vi "ControlProgram.vi"() -> ()   [LabVIEW 2017]
uses:
  C:/Users/laserpc/Desktop/Luis Alarcon/StepByStep/Thorlabs.MotionControl.Controls.dll
  Thorlabs.MotionControl.Controls.dll
panel:
  in  "KCubeInertialMotorControl":refnum<k24>(container)
  in  "stop 2":bool
  in  "SerialNumber":string="97000098"
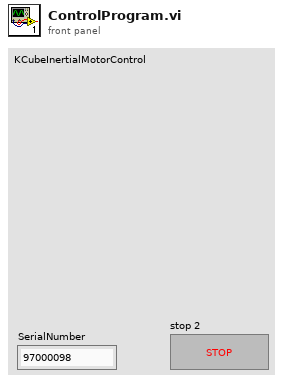
[diagram p1: front panel]
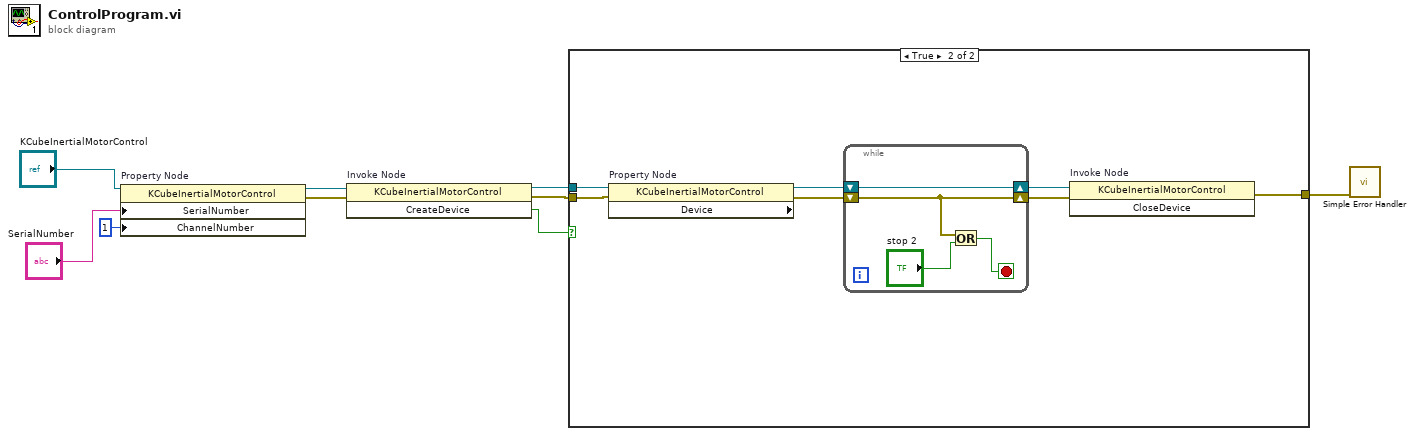
[diagram p0: block diagram]
diagram:
  n1 = property on="Property Node" class="KCubeInertialMotorControl"(reference="KCubeInertialMotorControl", "SerialNumber"="SerialNumber", "ChannelNumber"=1) -> (reference out=w8:refnum<k24>, error out=w5:errorcluster)  [unwired: 1 in]
  n2 = invoke on="Invoke Node" class="KCubeInertialMotorControl" method="CreateDevice"(reference=w8, error in=w5) -> (reference out=w7:refnum<k24>, error out=w2:errorcluster, "CreateDevice"=w3:bool)  [unwired: 1 in]
  n3 = case shown="True" w3 {
    tunnel: w7 -> [_ w17]
    tunnel: [w10 w16] -> w4
    tunnel: w2 -> [w10 w11]
    frame False {
    }
    frame True {
      n4 = property on="Property Node" class="KCubeInertialMotorControl" props=["Device"](reference=w17, error in=w11) -> (reference out=w15:refnum<k24>, error out=w14:errorcluster)  [unwired: 1 out]
      n5 = while {
        shift-right: [w20] -> w13
        shift-left: w14 -> [w20]
        shift-right: [w21] -> w12
        shift-left: w15 -> [w21]
        stop <- w18 stop-if-true
        n6 = Or(x=w20, y="stop 2") -> (x .or. y?=w18:bool)
      }
      n7 = invoke on="Invoke Node" class="KCubeInertialMotorControl" method="CloseDevice"(reference=w12, error in=w13) -> (error out=w16:errorcluster)  [unwired: 1 in, 2 out]
    }
  }
  n8 = call <vilib>:"Simple Error Handler.vi"("error in (no error)"=w4) -> ()  [unwired: 4 in, 5 out]
